vi "Init DAQmx Event.vi"(8 "error in (no error)":errorcluster, 11 "DAQmxAI in":refnum<class "DAQmxAI.lvclass">) -> (0 "error out":errorcluster, 3 "DAQmxAI out":refnum<class "DAQmxAI.lvclass">, 4 "Event Reg":refnum<event-registration>)   [LabVIEW 2020, in "VolatusDAQ.lvlib" / "DAQmxAI.lvclass"]
uses:
  DAQmxAI.lvclass
  DAQmxAI.lvclass/DAQmxAI.ctl
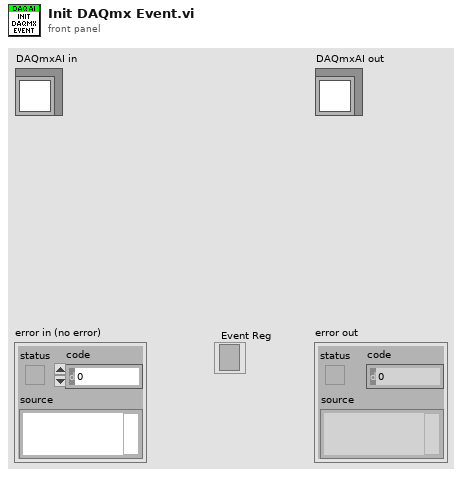
[diagram p1: front panel]
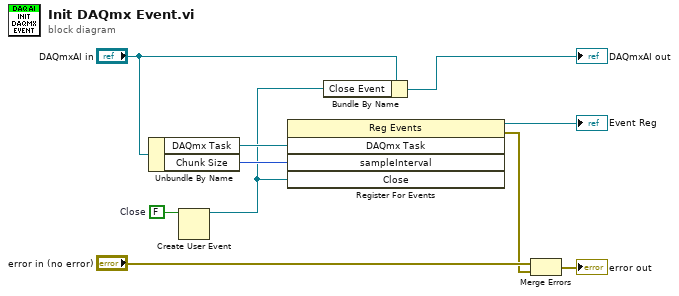
[diagram p0: block diagram]
diagram:
  w6 = FALSE  # Close
  n1 = Unbundle By Name("DAQmxAI in") -> ("DAQmx Task"=w9:refnum<k21>, "Chunk Size"=w7:i32)
  n2 = Create User Event(user event datatype=w6) -> (user event=w1:refnum<user-event>)  [unwired: 1 in, 1 out]
  n3 = register-events(w9, w7, w1) -> (reference out=→"Event Reg":refnum<event-registration>, error out=w3:errorcluster)  [unwired: 2 in]
  n4 = Bundle By Name(cluster="DAQmxAI in", "Close Event"=w1) -> (→"DAQmxAI out":refnum<class "DAQmxAI.lvclass">)
  n5 = Merge Errors("error in (no error)", w3) -> (→"error out":errorcluster)
